vi "_Read RT Table.vi"(4 "error in (no error)":errorcluster, 6 "key":string) -> (0 "error out":errorcluster, 1 "Table":dbl[][](array[numeric]))   [LabVIEW 2012]
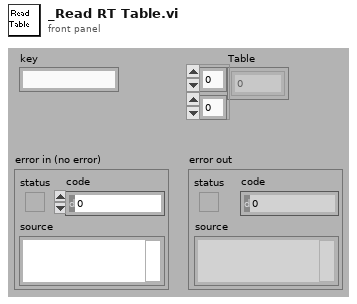
[diagram p1: front panel]
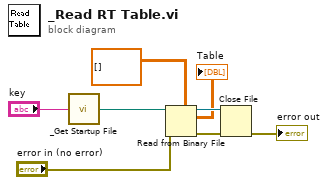
[diagram p0: block diagram]
diagram:
  n1 = call "_Get Startup File.vi"("FileName"="key") -> ("FilePath"=w2:path)
  n2 = Read from Binary File(5:dbl[][] [], 8:"error in (no error)", 11:w2) -> (0:w7:errorcluster, 2:→"Table":dbl[][], 3:w6:refnum<file>)  [unwired: 4 out]
  n3 = Close File(refnum=w6, error in=w7) -> (error out=→"error out":errorcluster)  [unwired: 1 out]
